vi "Event Is Nested.vi"(10 "Alias":string, 11 "Base Queue jettl in":refnum<class "Base Queue jettl.lvclass">) -> (2 "Event Is Nested?":bool, 3 "Base Queue jettl out":refnum<class "Base Queue jettl.lvclass">)   [LabVIEW 2021, in "jettl.lvlib" / "Base Queue jettl.lvlib" / "Base Queue jettl.lvclass"]
uses:
  Base Queue jettl.lvclass
  Base Queue jettl.lvclass/Base Queue jettl.ctl
  Queue Mailbox/Queue Mailbox.lvlib
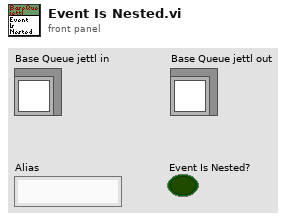
[diagram p1: front panel]
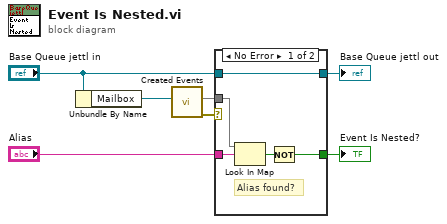
[diagram p0: block diagram]
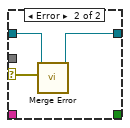
[diagram p2: hidden frame]
diagram:
  n1 = Unbundle By Name("Base Queue jettl in") -> ("Mailbox"=w5:refnum<data-value>)
  n2 = call "Created Events.vi"("Queue Mailbox"=w5) -> ("error out"=w1:errorcluster, "Event"=w4:map{string, refnum<data-value>})  [unwired: 9 in]
  n3 = case shown="No Error" w1 {
    selector: w1 -> [_ w13]
    tunnel: [w11 _] -> w7
    tunnel: "Alias" -> [w10 _]
    tunnel: w4 -> [w9 _]
    tunnel: "Base Queue jettl in" -> [w8 w15]
    tunnel: [w8 w14] -> w2
    frame No Error {
      # "Alias found?"
      n4 = Look In Map(map=w9, key=w10) -> (key not found?=w12:bool)  [unwired: 1 in, 1 out]
      n5 = Not(x=w12) -> (.not. x?=w11:bool)
    }
    frame Error {
      n6 = call-dynamic "Merge Error.vi"("Error"=w13, "Base Queue jettl in"=w15) -> ("Base Queue jettl out"=w14:refnum<class "Base Queue jettl.lvclass">)  [unwired: 9 in]
    }
  }
  "Event Is Nested?" <- w7
  "Base Queue jettl out" <- w2
